vi "power_meter.vi"() -> (2 "power_chart_01_mW":dbl(graph))   [LabVIEW 2014]
uses:
  <vilib>/Platform/TimedLoop/XDataNode/timing_clust.ctl
  <vilib>/Platform/TimedLoop/XDataNode/nitl_modes.ctl
  <vilib>/Platform/TimedLoop/XDataNode/wakeup.ctl
  <vilib>/platform/TimedLoop/XDataNode/XDataNode.xnode
  <vilib>/Platform/TimedLoop/XDataNode/XDNodeRunTimeDep.lvlib
panel:
  out "ratio":dbl caption="Ratio P2/P1 :" format="%.3f"
  in  "clear_plots":bool
  out "power_chart_02_mW":dbl(graph)
  in  "stop":bool
  # "P1: Laser Power after the dichroic"
  # "Laser power :"
  # "mW"
  # "P2: Laser Power in the sample holder"
  # "Laser power :"
  # "mW"
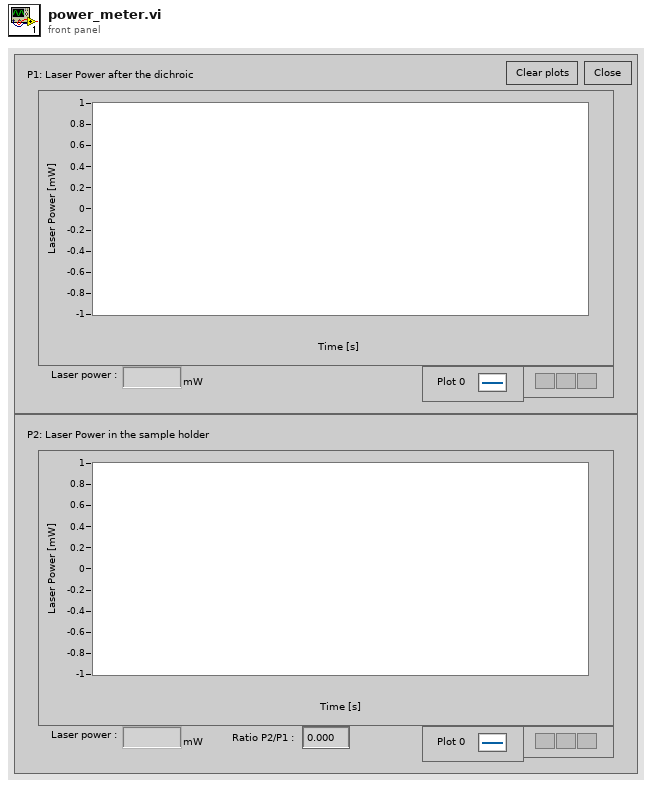
[diagram p1: front panel]
types:
  T1 = typedef "XDNodeRunTimeDep.lvlib/timing_clust.ctl" = cluster{"Expected End [f-1]":u64, "Actual End [f-1]":u64, "Finished Late? [f-1]":bool, "Expected End [i-1]":u64, "Actual End [i-1]":u64, "Finished Late? [i-1]":bool, "Expected Start [i]":u64, "Actual Start [i]":u64, "Expected Start [f]":u64, "Actual Start [f]":u64, "Source Name":string, "Structure Name":string, "Period":i64, "Deadline":i64, "Offset":i64, "Start":i64, "Priority":i32, "Timeout":i32, "Mode":T2, "Wakeup Reason":T3, "Error":errorcluster, "Source Type":string, "Secondary Source Type":string, "Global End Time":u64, "Global Start Time":u64, "Frame Duration":u64, "Iteration Duration":u64, "Assigned CPU":i32, "I/O Scan Engine Mode":u32}
  T2 = typedef "XDNodeRunTimeDep.lvlib/nitl_modes.ctl" = enum32{"No Change", "Process missed periods, maintain original phase", "Discard missed periods, maintain original phase", "Process missed periods, ignore original phase", "Discard missed periods, ignore original phase"}
  T3 = typedef "XDNodeRunTimeDep.lvlib/wakeup.ctl" = enum32{"Normal", "Aborted", "Asynchronous wakeup", "Timing source error", "Timed loop error", "Timeout"}
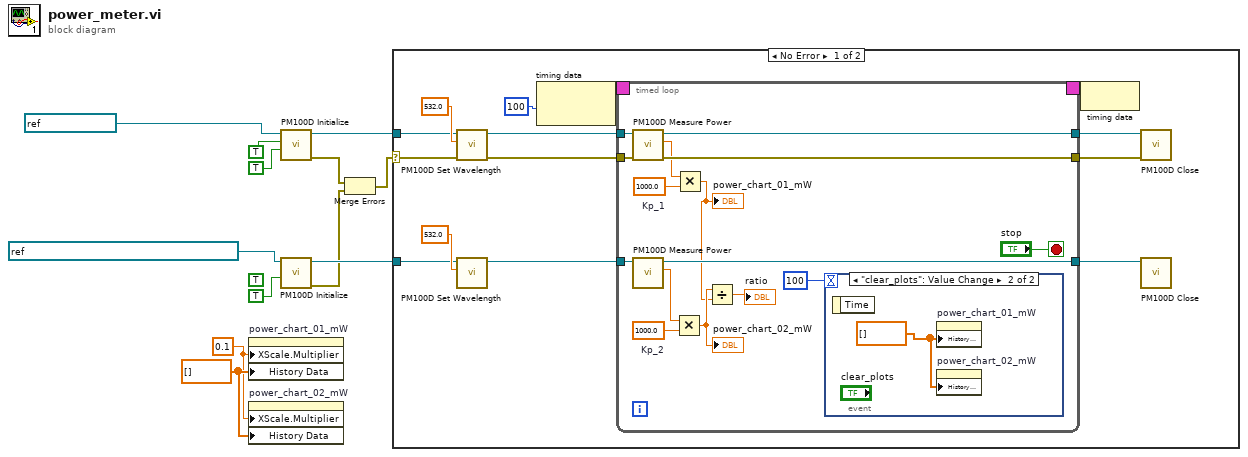
[diagram p0: block diagram]
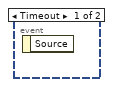
[diagram p2: hidden frame]
diagram:
  (unwired) TRUE ("ID Query (Do Query)")
  w2 = dbl[] [] ("History Data")
  w1 = 0.1 ("X Scale.Offset and Multiplier:Multiplier")
  n1 = property on="power_chart_01_mW" class="WFChart (strict)"("XScale.Multiplier"=w1, "History Data"=w2) -> ()  [unwired: 2 in, 2 out]
  n2 = property on="power_chart_02_mW" class="WFChart (strict)"("XScale.Multiplier"=w1, "History Data"=w2) -> ()  [unwired: 2 in, 2 out]
  n3 = call <instrlib>:"PM100D Initialize.vi"("Reset Device (Reset Device)"=TRUE ("ID Query (Do Query)"), "ID Query (Do Query)"=TRUE, "resource name"=refnum<visa-resource-name> "PowerMeter") -> ("error out"=w4:errorcluster, "instrument handle out"=w10:refnum<visa-resource-name>)  [unwired: 7 in]
  n4 = call <instrlib>:"PM100D Initialize.vi"("Reset Device (Reset Device)"=TRUE ("ID Query (Do Query)"), "resource name"=refnum<visa-resource-name> "USB0::0x1313::0x8078::P0007815::INSTR") -> ("error out"=w5:errorcluster, "instrument handle out"=w6:refnum<visa-resource-name>)  [unwired: 8 in]
  n5 = Merge Errors(w4, w5) -> (w3:errorcluster)
  n6 = case shown="No Error" w3 {
    selector: w3 -> [w20 _]
    tunnel: w10 -> [w19 _]
    tunnel: w6 -> [w15 _]
    frame No Error {
      n7 = call <instrlib>:"PM100D Set Wavelength.vi"("error in (no error)"=w20, "Wavelength (0.0)"=532.0, "instrument handle"=w19) -> ("error out"=w17:errorcluster, "instrument handle out"=w18:refnum<visa-resource-name>)  [unwired: 7 in]
      n8 = call <instrlib>:"PM100D Set Wavelength.vi"("Wavelength (0.0)"=532.0, "instrument handle"=w15) -> ("instrument handle out"=w14:refnum<visa-resource-name>)  [unwired: 8 in, 1 out]
      n9 = node-c288(i64 100 ("Period")) -> (w26:T1)
      n10 = timed-loop {
        timing: w26 -> [_]
        timing-out: [_] -> w25
        tunnel: w18 -> [w41]
        tunnel: [w40] -> w23
        tunnel: w17 -> [w39]
        tunnel: [w38] -> w22
        tunnel: w14 -> [w33]
        tunnel: [w32] -> w13
        stop <- "stop" stop-if-true
        w34 = 1000.0  # Kp_2
        w36 = 1000.0  # Kp_1
        n11 = call <instrlib>:"PM100D Measure Power.vi"("error in (no error)"=w39, "instrument handle"=w41) -> ("error out"=w38:errorcluster, "Power"=w37:dbl, "instrument handle out"=w40:refnum<visa-resource-name>)  [unwired: 7 in]
        n12 = call <instrlib>:"PM100D Measure Power.vi"("instrument handle"=w33) -> ("Power"=w31:dbl, "instrument handle out"=w32:refnum<visa-resource-name>)  [unwired: 8 in, 1 out]
        n13 = Multiply(x=w31, y=w34) -> (x*y=w28:dbl)
        "power_chart_02_mW" <- w28
        n14 = Multiply(x=w37, y=w36) -> (x*y=w27:dbl)
        "power_chart_01_mW" <- w27
        n15 = Divide(x=w28, y=w27) -> (x/y=→"ratio":dbl)
        n16 = event shown="[1] \"clear_plots\": Value Change" {
          selector: _ -> [_ _]
          dyn-events: _ -> [_ _]
          timeout: 100 -> [_ _]
          event Timeout {
            n17 = event-data() -> ()  [unwired: 1 in, 1 out]
          }
          event "clear_plots": Value Change {
            w42 = dbl[] [] ("History Data")
            n18 = event-data() -> ()  [unwired: 1 in, 1 out]
            n19 = property on="power_chart_01_mW" class="WFChart (strict)"("History Data"=w42) -> ()  [unwired: 2 in, 2 out]
            n20 = property on="power_chart_02_mW" class="WFChart (strict)"("History Data"=w42) -> ()  [unwired: 2 in, 2 out]
          }
        }
      }
      n21 = node-c288(w25) -> ()
      n22 = call <instrlib>:"PM100D Close.vi"("error in (no error)"=w22, "instrument handle"=w23) -> ()  [unwired: 9 in, 1 out]
      n23 = call <instrlib>:"PM100D Close.vi"("instrument handle"=w13) -> ()  [unwired: 10 in, 1 out]
    }
    frame Error {
    }
  }
